vi "7HP_Convert serial string to Eng vals.vi"(0 "Serial buffer string (excluding FrameChar)":string) -> (9 "All vals":sgl[](array[numeric]), 11 "ANN output vector":sgl[](array[numeric]), 12 "Pressures":sgl[][](graph), 13 "Gyration vector (deg / s)":sgl[](array[numeric]), 14 "External thermistor temperature (deg C)":sgl, 15 "Atmospheric pressure (mbar)":sgl, 17 "Env. sensor die temperature (deg C)":sgl, 18 "Relative humidity (%)":sgl, 19 "Acceleration vector (g)":sgl[](array[numeric]))   [LabVIEW 2021]
panel:
  # "||U|| (m/s)"
  # "Pitch (deg)"
  # "Yaw (deg)"
  # "U (m/s)"
  # "V (m/s)"
  # "W (m/s)"
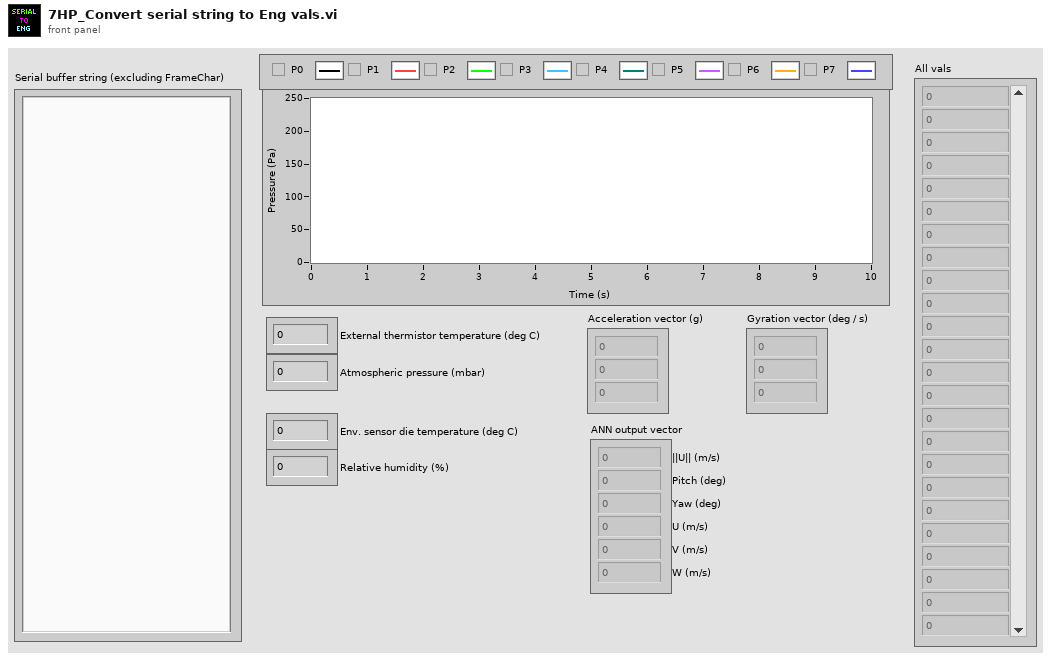
[diagram p1: front panel]
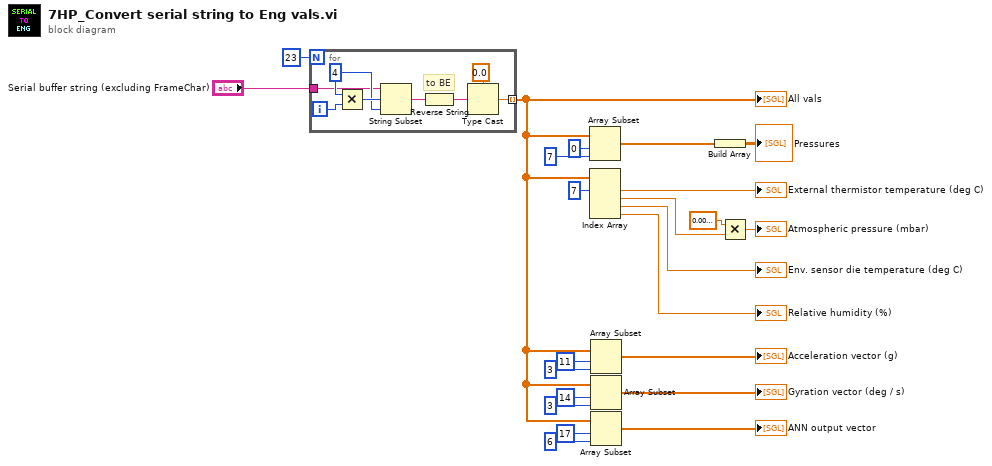
[diagram p0: block diagram]
diagram:
  n1 = for {
    N: 23 -> [_]
    tunnel: [w25] -> w2 mode=indexing
    tunnel: "Serial buffer string (excluding FrameChar)" -> [w24]
    i -> [w31]
    w29 = 4 ("x")
    # "to BE"
    n2 = Multiply(x=w29, y=w31) -> (x*y=w30:i32)
    n3 = String Subset(string=w24, offset (0)=w30, length (rest)=w29) -> (substring=w28:string)
    n4 = Reverse String(1:w28) -> (0:w27:string)
    n5 = Type Cast(type=sgl 0.0 ("byte count"), x=w27) -> (*(type *) &x=w25:sgl)
  }
  "All vals" <- w2
  n6 = Array Subset(array=w2, index=0, length=7) -> (w10:sgl[])
  n7 = Index Array(array=w2, index #1=7 ("index")) -> (element #1=→"External thermistor temperature (deg C)":sgl, element #2=w7:sgl, element #3=→"Env. sensor die temperature (deg C)":sgl, element #4=→"Relative humidity (%)":sgl)  [unwired: 3 in]
  n8 = Array Subset(array=w2, index=11, length=3) -> (→"Acceleration vector (g)":sgl[])
  n9 = Array Subset(array=w2, index=14, length=3) -> (→"Gyration vector (deg / s)":sgl[])
  n10 = Array Subset(array=w2, index=17, length=6) -> (→"ANN output vector":sgl[])
  n11 = Build Array(w10) -> (→"Pressures":sgl[][])
  n12 = Multiply(x=sgl 0.01, y=w7) -> (x*y=→"Atmospheric pressure (mbar)":sgl)
